vi "Creat_Queue_Message.vi"(11 "Message_Queue":T1) -> (3 "Message_Queue Out":T1)   [LabVIEW 2014, in "Queue_Library.lvlib"]
uses:
  Queue_Library.lvlib
  QMH_Function_vi/Control/Queue_Message_TypeDef.ctl
  TypeDef.ctl
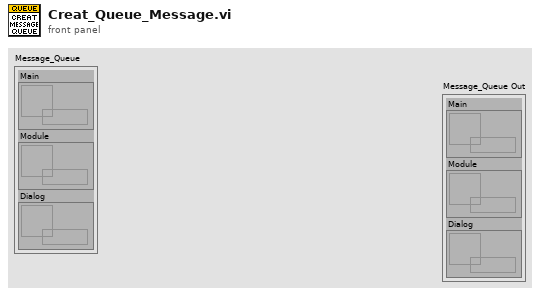
[diagram p1: front panel]
types:
  T1 = typedef "Queue_Message_TypeDef.ctl" = cluster{"Main":refnum<queue>, "Module":refnum<queue>, "Dialog":refnum<queue>}
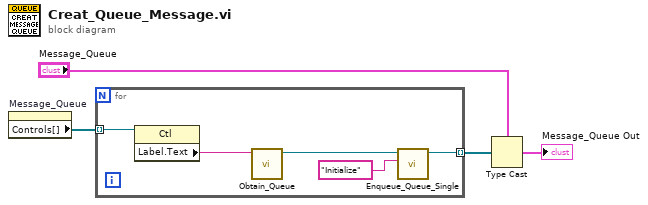
[diagram p0: block diagram]
diagram:
  n1 = property on="Message_Queue" class="Clust (strict)"() -> ("Controls[]"=w4:refnum<vi>[])  [unwired: 2 in, 2 out]
  n2 = for {
    tunnel: w4 -> [w7] mode=indexing
    tunnel: [w5] -> w3 mode=indexing
    n3 = property class="Ctl"(reference=w7) -> ("Label.Text"=w6:string)  [unwired: 1 in, 2 out]
    n4 = call "Obtain_Queue.vi"("Name"=w6) -> ("queue out"=w9:refnum<queue>)  [unwired: 9 in, 1 out]
    n5 = call "Enqueue_Queue_Single.vi"("Command"="Initialize", "queue In"=w9) -> ("queue Out"=w5:refnum<queue>)  [unwired: 8 in, 1 out]
  }
  n6 = Type Cast(type="Message_Queue", x=w3) -> (*(type *) &x=→"Message_Queue Out":T1)
